vi "Parallel CR write.vi"(0 "-Strobe":enum16{"FALSE", "TRUE", "No Change"}(ring)=enum."No Change", 1 "-AutoLF":enum16{"FALSE", "TRUE", "No Change"}(ring)=enum."No Change", 2 "-Init":enum16{"FALSE", "TRUE", "No Change"}(ring)=enum."No Change", 3 "-Select In":enum16{"FALSE", "TRUE", "No Change"}(ring)=enum."No Change", 4 "Port Base Address":u32) -> (5 "Register Value Written":u8)   [LabVIEW 2014]
doc: "Write to Control Register of Parallel Port\nThis VI determines a new control register configuration for a parallel port and writes it. The four named bits may be set low, set high or left unchanged (the default). The Port Base Address should be the _base_ address; from there the VI gets the address of the control register itself.\nNote that this sets the output at the connector to the requested state. You need not worry about the fact that for some bits the register is actually inverted relative to the output. This is separate from the fact that they may be 'active low' (which they all are under normal use). The output is what was actually written to the register, and will reflect this wierdness.\nThis VI uses the National Instruments AccessHW package to access the registers under Windows XP."
uses:
  <vilib>/Platform/portaccess.llb/In Port8.vi
  <vilib>/Platform/portaccess.llb/Out Port8.vi
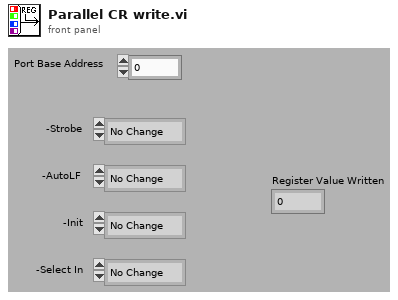
[diagram p1: front panel]
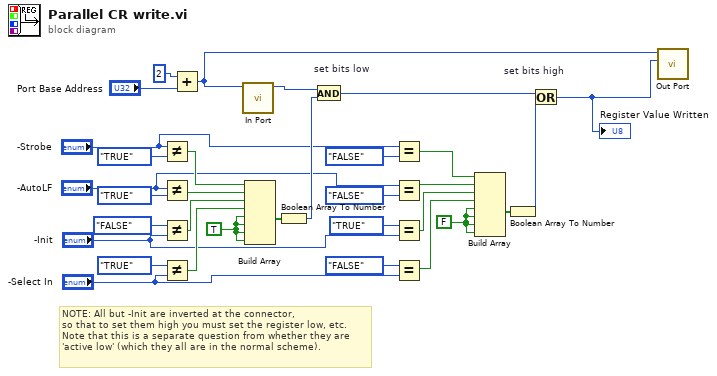
[diagram p0: block diagram]
diagram:
  w21 = FALSE ("element")
  w28 = TRUE ("element")
  # "NOTE: All but -Init are inverted at the connector,\nso that to set them high you must set the register low, etc.\nNote that this is a separate question from whether they are\n'active low' (which they all are in the normal scheme)."
  n1 = Not Equal?(x="-Strobe", y=enum16{"FALSE", "TRUE", "No Change"}."TRUE") -> (x != y?=w30:bool)
  n2 = Not Equal?(x="-AutoLF", y=enum16{"FALSE", "TRUE", "No Change"}."TRUE") -> (x != y?=w24:bool)
  n3 = Not Equal?(x=enum16{"FALSE", "TRUE", "No Change"}."FALSE", y="-Init") -> (x != y?=w23:bool)
  n4 = Not Equal?(x=enum16{"FALSE", "TRUE", "No Change"}."TRUE", y="-Select In") -> (x != y?=w29:bool)
  n5 = Add(x=u32 2, y="Port Base Address") -> (x+y=w2:u32)
  n6 = call-poly <vilib>:"In Port.vi"("address"=w2) -> ("data read"=w3:i8)  [unwired: 7 in, 1 out]
  n7 = Build Array(w30, w24, w23, w29, w28, w28, w28, w28) -> (w27:bool[])
  n8 = Boolean Array To Number(Boolean array=w27) -> (number=w26:u32)
  n9 = And "set bits low"(x=w3, y=w26) -> (x .and. y?=w14:u32)
  n10 = Equal?(x="-Strobe", y=enum16{"FALSE", "TRUE", "No Change"}."FALSE") -> (x = y?=w18:bool)
  n11 = Equal?(x="-AutoLF", y=enum16{"FALSE", "TRUE", "No Change"}."FALSE") -> (x = y?=w17:bool)
  n12 = Equal?(x=enum16{"FALSE", "TRUE", "No Change"}."TRUE", y="-Init") -> (x = y?=w16:bool)
  n13 = Equal?(x=enum16{"FALSE", "TRUE", "No Change"}."FALSE", y="-Select In") -> (x = y?=w15:bool)
  n14 = Build Array(w18, w17, w16, w15, w21, w21, w21, w21) -> (w20:bool[])
  n15 = Boolean Array To Number(Boolean array=w20) -> (number=w19:u32)
  n16 = Or "set bits high"(x=w14, y=w19) -> (x .or. y?=w1:u32)
  "Register Value Written" <- w1
  n17 = call-poly <vilib>:"Out Port.vi"("write value"=w1, "address"=w2) -> ()  [unwired: 7 in, 1 out]
